vi "get limits.vi"(10 "External Supply?":bool=TRUE, 11 "Channel #":T1) -> (3 "output cluster":T2)   [LabVIEW 2015, in "NI PXI-4110 Programmable Power Supply Custom Device.lvlib"]
uses:
  NI PXI-4110 Programmable Power Supply Custom Device.lvlib
  4110_Channel #.ctl
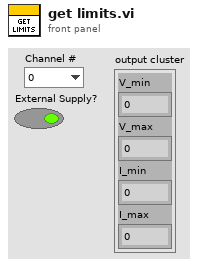
[diagram p1: front panel]
types:
  T1 = typedef "NI PXI-4110 Programmable Power Supply Custom Device.lvlib/4110_Channel #.ctl" = enum16{"0", "1", "2"}
  T2 = cluster{"V_min":dbl, "V_max":dbl, "I_min":dbl, "I_max":dbl}
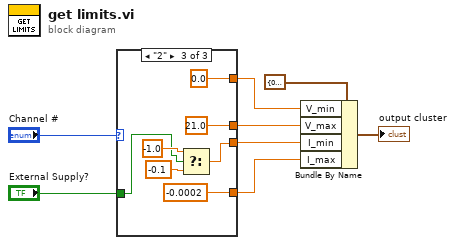
[diagram p0: block diagram]
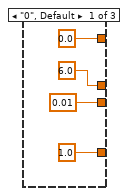
[diagram p2: hidden frame]
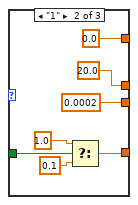
[diagram p3: hidden frame]
diagram:
  n1 = case shown="\"2\"" "Channel #" {
    tunnel: [0.0 ("V_min") 0.0 ("V_min") 0.0 ("V_min")] -> w3
    tunnel: [6.0 ("V_min") 20.0 ("V_min") 21.0 ("V_min")] -> w4
    tunnel: [0.01 ("V_min") 0.0002 ("V_min") w21] -> w5
    tunnel: [1.0 ("V_min") w13 -0.0002 ("V_min")] -> w6
    tunnel: "External Supply?" -> [_ w16 w20]
    frame "0", Default {
    }
    frame "1" {
      n2 = Select(t=1.0, s=w16, f=0.1 ("V_min")) -> (s? t:f=w13:dbl)
    }
    frame "2" {
      n3 = Select(t=-1.0, s=w20, f=-0.1 ("V_min")) -> (s? t:f=w21:dbl)
    }
  }
  n4 = Bundle By Name(cluster=T2 {"V_min"=0.0, "V_max"=0.0, "I_min"=0.0, "I_max"=0.0} ("output cluster"), "V_min"=w3, "V_max"=w4, "I_min"=w5, "I_max"=w6) -> (→"output cluster":T2)
